vi "SetAngle.vi"(8 "error in (no error)":errorcluster, 11 "Cargo in":refnum<class "Cargo.lvclass">) -> (0 "error out":errorcluster, 3 "Cargo out":refnum<class "Cargo.lvclass">)   [LabVIEW 2018]
uses:
  Cargo.lvclass
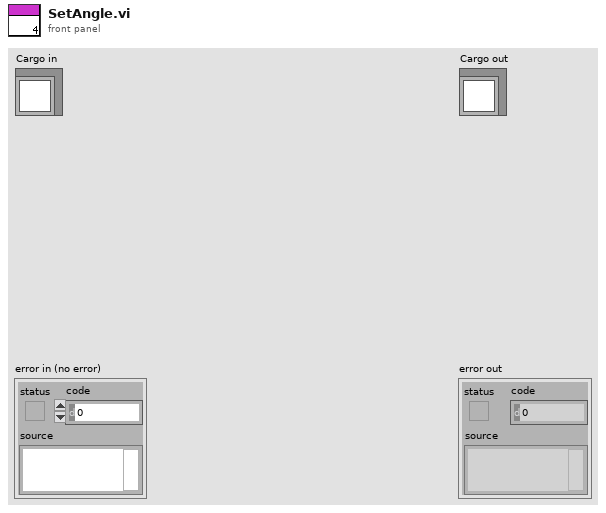
[diagram p1: front panel]
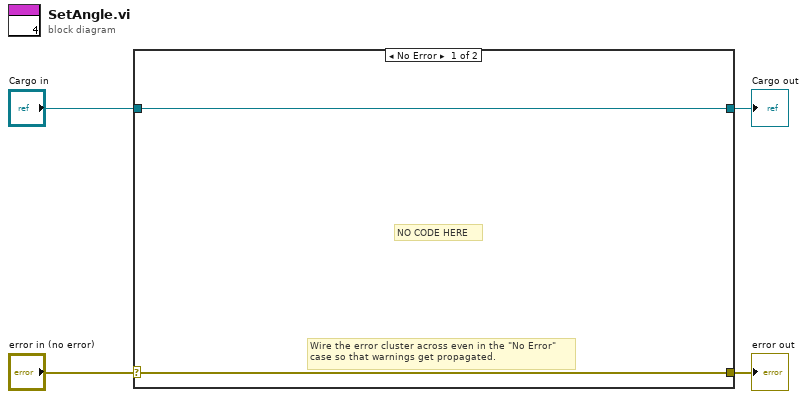
[diagram p0: block diagram]
diagram:
  n1 = case shown="No Error" "error in (no error)" {
    selector: "error in (no error)" -> [w5 w8]
    tunnel: [w5 w8] -> w3
    tunnel: [w6 w7] -> w1
    tunnel: "Cargo in" -> [w6 w7]
    frame No Error {
      # "NO CODE HERE"
      # "Wire the error cluster across even in the \"No Error\"\ncase so that warnings get propagated."
    }
    frame Error {
    }
  }
  "error out" <- w3
  "Cargo out" <- w1
